vi "initAudio.vi"(8 "error in (no error)":errorcluster, 9 "Physical channel A for audio input":tag, 10 "Samples per\nacquisition chunk":i32, 11 "Audio sample rate (Hz)":i64) -> (0 "error out":errorcluster, 2 "SampClk.Rate":dbl, 3 "Refnum out":refnum<k21>)   [LabVIEW 2017]
uses:
  <vilib>/DAQmx/create/channels.llb/DAQmx Create Channel (AI-Voltage-Basic).vi
  <vilib>/DAQmx/configure/timing.llb/DAQmx Timing (Sample Clock).vi
  <resource>/objmgr/daqmx.rc
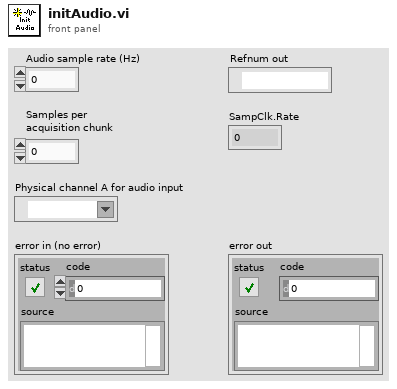
[diagram p1: front panel]
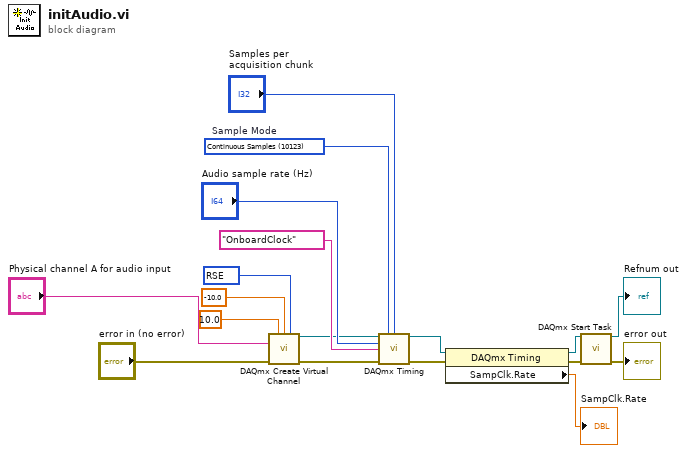
[diagram p0: block diagram]
diagram:
  w5 = 10083 items=["default"=-1, "RSE"=10083, "NRSE"=10078, "Differential"=10106, "Pseudodifferential"=12529] ("Terminal Configuration")
  w1 = 10123 items=["Finite Samples"=10178, "Continuous Samples"=10123, "Hardware Timed Single Point"=12522]  # Sample Mode
  n1 = call-poly <vilib>:"DAQmx Create Virtual Channel.vi"("maximum value"=10.0 ("Max Voltage"), "minimum value"=-10.0 ("Min Voltage"), "input terminal configuration"=w5, "physical channels"="Physical channel A for audio input", "error in"="error in (no error)") -> ("task out"=w3:refnum<k21>, "error out"=w2:errorcluster)  [unwired: 9 in]
  n2 = call-poly <vilib>:"DAQmx Timing.vi"("task/channels in"=w3, "sample mode"=w1, "samples per channel"="Samples per\nacquisition chunk", "rate"="Audio sample rate (Hz)", "source"=tag "OnboardClock" ("Sample Clock Source"), "error in"=w2) -> ("task out"=w11:refnum<k21>, "error out"=w12:errorcluster)  [unwired: 8 in]
  n3 = property class="DAQmx Timing"(reference=w11, error in=w12) -> (reference out=w14:refnum<k21>, error out=w15:errorcluster, "SampClk.Rate"=→"SampClk.Rate":dbl)
  n4 = call <vilib>:"DAQmx Start Task.vi"("task/channels in"=w14, "error in"=w15) -> ("task out"=→"Refnum out":refnum<k21>, "error out"=→"error out":errorcluster)  [unwired: 12 in]
